vi "Server_Refresh Log Data.vi"(8 "error in":errorcluster, 11 "Index":i32) -> (0 "error out":errorcluster, 2 "Data Query List":string[][](array[string]), 3 "Data":waveform(dbl)[](array[waveform]))   [LabVIEW 2018, in "Cloud Server.lvlib"]
uses:
  Cloud Server.lvlib
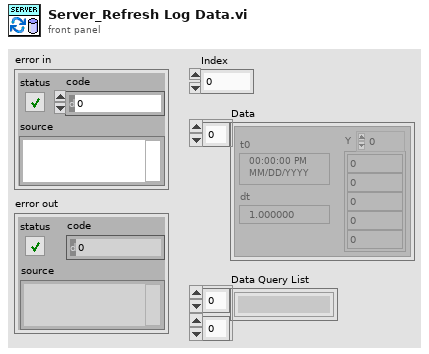
[diagram p1: front panel]
types:
  T1 = typedef "Cloud Server.lvlib/Server_Connection Properties.ctl" = cluster{"User Data":T2, "Data":waveform(dbl)}
  T2 = typedef "User Data.ctl" = cluster{"Name":string, "Email":string, "Phone Number":string, "User Picture":u32[][], "Last Login Time":timestamp}
  T3 = typedef "Data File Format.ctl" = cluster{"Data":waveform(dbl), "Abnormal?":bool, "Measure Time":timestamp, "User Name":string}
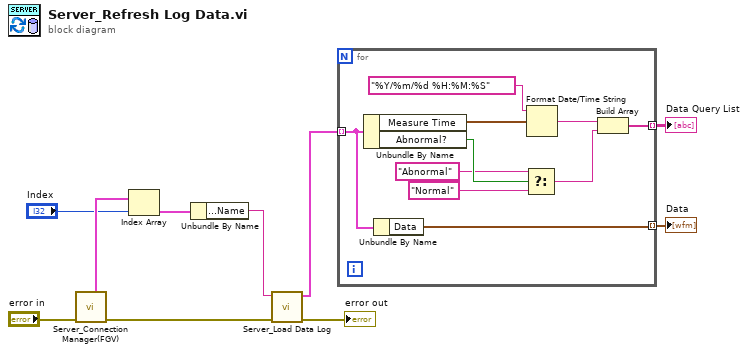
[diagram p0: block diagram]
diagram:
  n1 = call "Server_Connection Manager(FGV).vi"("error in"="error in") -> ("error out"=w6:errorcluster, "All Connection Properties"=w10:T1[])  [unwired: 6 in, 3 out]
  n2 = Index Array(array=w10, index="Index") -> (element=w7:T1)
  n3 = Unbundle By Name(w7) -> ("User Data.Name"=w5:string)
  n4 = call "Server_Load Data Log.vi"("error in"=w6, "User Name"=w5) -> ("error out"=→"error out":errorcluster, "Log Data"=w4:T3[])  [unwired: 8 in]
  n5 = for {
    tunnel: w4 -> [w12] mode=indexing
    tunnel: [w13] -> w2 mode=indexing
    tunnel: [w11] -> w3 mode=indexing
    n6 = Unbundle By Name(w12) -> ("Measure Time"=w19:timestamp, "Abnormal?"=w17:bool)
    n7 = Unbundle By Name(w12) -> ("Data"=w11:waveform(dbl))
    n8 = Select(t="Abnormal" ("time format string (%c)"), s=w17, f="Normal" ("time format string (%c)")) -> (s? t:f=w14:string)
    n9 = Format Date/Time String(time format string (%c)="%Y/%m/%d %H:%M:%S", seconds (now)=w19) -> (date/time string=w18:string)  [unwired: 1 in]
    n10 = Build Array(w18, w14) -> (w13:string[])
  }
  "Data" <- w3
  "Data Query List" <- w2
